vi "Generate View Event.vi"(8 "error in (no error)":errorcluster, 10 "Event Data":refnum<class "Event.lvclass">, 11 "View in":refnum<class "View.lvclass">) -> (0 "error out":errorcluster, 3 "View out":refnum<class "View.lvclass">)   [LabVIEW 2023, in "MVC Actors.lvlib" / "View.lvclass"]
doc: "This method generates/fires the Event wired to the input. Firing an event checks if the view is paused or \"Receive Only\" . This event will not be broadcast to other Views.\n\n<b>IMPORTANT</b> - Only call this method directly (i.e. without sending the corresponding message) only within the View methods. From helper loops send the corresponding message to self by calling the suitable send method. This is to make sure your View works with up-to-date settings."
uses:
  View.lvclass
  Event/Event.lvclass
  View.lvclass/View.ctl
  properties/Read Controller Actor Enqueuer.vi
  properties/Read Paused.vi
  properties/Read Receive Only.vi
  <vilib>/ActorFramework/Message Enqueuer/Message Enqueuer.lvclass
  Controller Messages/Handle Event Msg/Handle Event Msg.lvclass
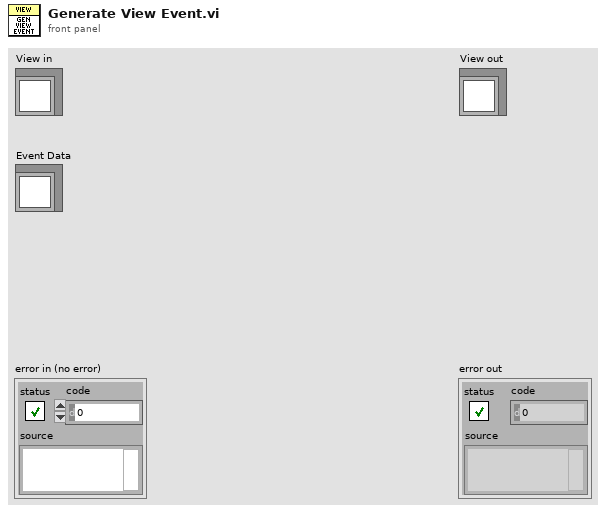
[diagram p1: front panel]
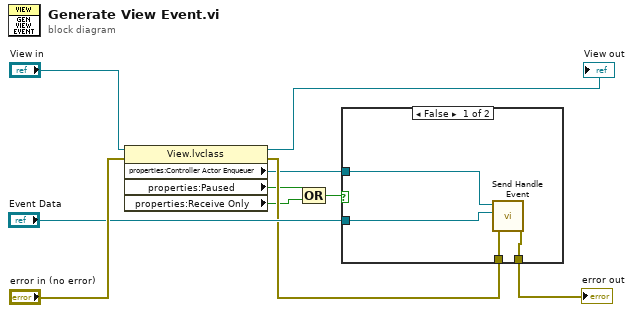
[diagram p0: block diagram]
diagram:
  n1 = property class="View.lvclass"(reference="View in", error in="error in (no error)") -> (reference out=→"View out":refnum<class "View.lvclass">, error out=w7:errorcluster, "properties:Controller Actor Enqueuer"=w5:refnum<class "Message Enqueuer.lvclass">, "properties:Paused"=w3:bool, "properties:Receive Only"=w2:bool)
  n2 = Compound Arithmetic op=OR(w3, w2) -> (w1:bool)
  n3 = case shown="False" w1 {
    tunnel: "Event Data" -> [w13 _]
    tunnel: w7 -> [w12 w15]
    tunnel: [w11 w15] -> w6
    tunnel: w5 -> [w14 _]
    frame False {
      n4 = call "Send Handle Event.vi"("error in (no error)"=w12, "Event Data"=w13, "Message Enqueuer in"=w14) -> ("error out"=w11:errorcluster)  [unwired: 7 in, 1 out]
    }
    frame True {
    }
  }
  "error out" <- w6
